vi "SignalProcessing Global.vi"() -> ()   [LabVIEW 2019, in "SignalProcessing.lvlib" / "SignalProcessing.lvclass"]
uses:
  SignalProcessing.lvclass
panel:
  in  "TestComplete writer endpoint 4":refnum<k21>
  in  "TestComplete writer endpoint 3":refnum<k21>
  in  "TestComplete writer endpoint 2":refnum<k21>
  in  "Station(SignalProcessing)":i32
  in  "TestComplete writer endpoint 1":refnum<k21>
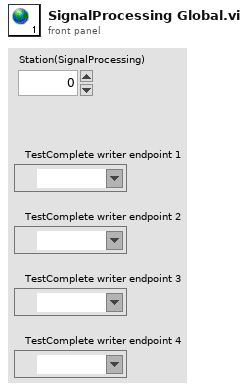
[diagram p1: front panel]
diagram:
